vi "Read Config File.vi"(8 "error in (no error)":errorcluster, 11 "SM EOL Station Actor in":refnum<class "PLC Sim Controller Actor.lvclass">) -> (0 "error out":errorcluster, 3 "SM EOL Station Actor out":refnum<class "PLC Sim Controller Actor.lvclass">)   [LabVIEW 2019, in "PLC Sim Controller Actor.lvlib" / "PLC Sim Controller Actor.lvclass"]
uses:
  PLC Sim Controller Actor.lvclass
  PLC Sim Controller Actor.lvclass/PLC Sim Controller Actor.ctl
  <vilib>/Utility/config.llb/Read Key (I32).vi
  <vilib>/Utility/config.llb/Read Key (String).vi
  <vilib>/Utility/config.llb/NI_LVConfig.lvlib
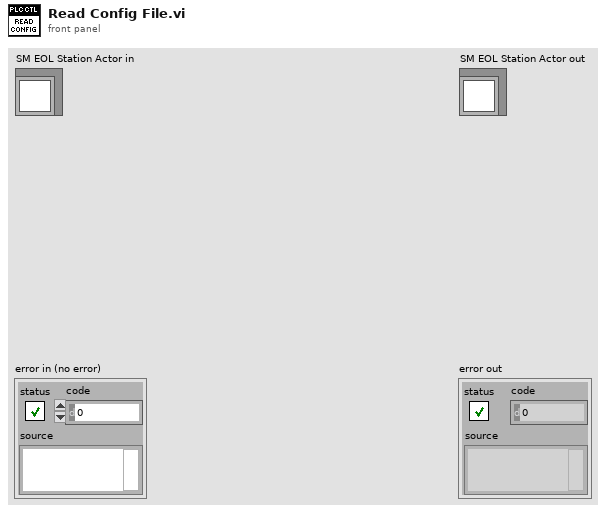
[diagram p1: front panel]
types:
  T1 = typedef "NI_LVConfig.lvlib/Config Data RefNum.ctl" = refnum<k1>
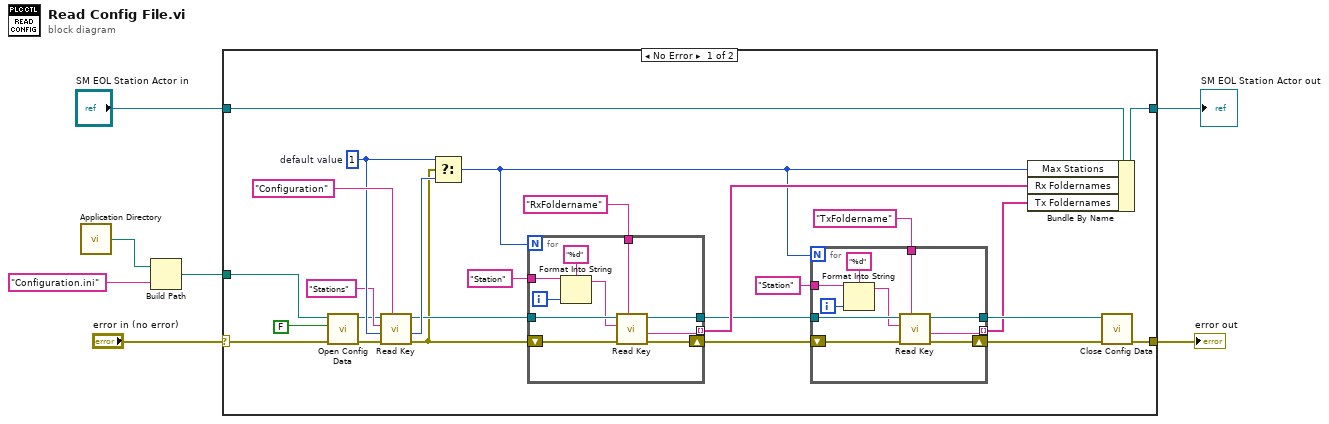
[diagram p0: block diagram]
diagram:
  n1 = call <vilib>:"Application Directory.vi"() -> ("Application Directory"=w1:path)
  n2 = Build Path(base path=w1, name or relative path="Configuration.ini") -> (appended path=w3:path)
  n3 = case shown="No Error" "error in (no error)" {
    selector: "error in (no error)" -> [w20 w54]
    tunnel: [w19 w54] -> w6
    tunnel: [w25 w53] -> w4
    tunnel: "SM EOL Station Actor in" -> [w9 w53]
    tunnel: w3 -> [w21 _]
    frame No Error {
      w30 = 1  # default value
      n4 = call <vilib>:"Open Config Data.vi"("error in (no error)"=w20, "create file if necessary (T)"=FALSE, "configuration file path"=w21) -> ("error out"=w27:errorcluster, "refnum"=w28:T1)  [unwired: 6 in, 1 out]
      n5 = call-poly <vilib>:"Read Key.vi"("section"="Configuration", "error in (no error)"=w27, "default value"=w30, "key"="Stations", "refnum"=w28) -> ("error out"=w23:errorcluster, "value"=w31:i32, "refnum out"=w24:T1)  [unwired: 3 in, 1 out]
      n6 = Select(t=w30, s=w23, f=w31) -> (s? t:f=w16:i32)
      n7 = for {
        N: w16 -> [_]
        tunnel: [w50] -> w22 mode=indexing
        shift-right: [w49] -> w15
        shift-left: w23 -> [w51]
        tunnel: w24 -> [w52]
        tunnel: [w48] -> w12
        tunnel: "Station" ("key") -> [w47]
        tunnel: "RxFoldername" ("section") -> [w43]
        i -> [w45]
        n8 = Format Into String(format string="%d", initial string=w47, w45) -> (resulting string=w44:string)  [unwired: 1 in, 1 out]
        n9 = call-poly <vilib>:"Read Key.vi"("section"=w43, "error in (no error)"=w51, "key"=w44, "refnum"=w52) -> ("error out"=w49:errorcluster, "value"=w50:string, "refnum out"=w48:T1)  [unwired: 4 in, 1 out]
      }
      n10 = for {
        N: w16 -> [_]
        tunnel: [w40] -> w8 mode=indexing
        shift-right: [w39] -> w11
        shift-left: w15 -> [w41]
        tunnel: w12 -> [w42]
        tunnel: [w38] -> w10
        tunnel: "Station" ("key") -> [w37]
        tunnel: "TxFoldername" ("section") -> [w33]
        i -> [w35]
        n11 = Format Into String(format string="%d", initial string=w37, w35) -> (resulting string=w34:string)  [unwired: 1 in, 1 out]
        n12 = call-poly <vilib>:"Read Key.vi"("section"=w33, "error in (no error)"=w41, "key"=w34, "refnum"=w42) -> ("error out"=w39:errorcluster, "value"=w40:string, "refnum out"=w38:T1)  [unwired: 4 in, 1 out]
      }
      n13 = Bundle By Name(cluster=w9, "Max Stations"=w16, "Rx Foldernames"=w22, "Tx Foldernames"=w8) -> (w25:refnum<class "PLC Sim Controller Actor.lvclass">)
      n14 = call <vilib>:"Close Config Data.vi"("error in (no error)"=w11, "refnum"=w10) -> ("error out"=w19:errorcluster)  [unwired: 8 in, 1 out]
    }
    frame Error {
    }
  }
  "error out" <- w6
  "SM EOL Station Actor out" <- w4
